vi "Send Command.vi"(7 "Config offset":u64 format="%x", 8 "error in (no error)":errorcluster, 9 "Command payload":u64 format="%x", 10 "Command number":T1, 11 "RP Instrument in":refnum<class "RP Instrument.lvclass">) -> (0 "error out":errorcluster, 3 "RP Instrument out":refnum<class "RP Instrument.lvclass">)   [LabVIEW 2024, in "RP Instrument.lvclass"]
uses:
  RP Instrument.lvclass
  RP Command.ctl
  RP Instrument.lvclass/RP Instrument.ctl
  RP Communicator/RP Communicator.lvclass
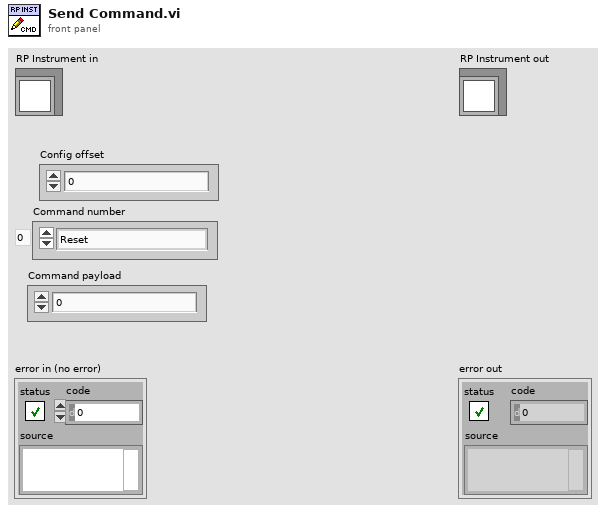
[diagram p1: front panel]
types:
  T1 = typedef "RP Command.ctl" = enum16{"Reset", "Read IDN", "Stop server", "Get status", "Get temperature", "Connect client", "Arm", "Software trigger", "Get whole buffer", "Get chunk", "System call", "Get config", "Set config", "Recieve data", "Recieve Calibartion", "Transmit data"}
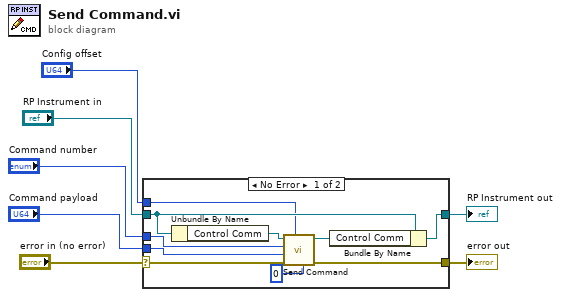
[diagram p0: block diagram]
diagram:
  n1 = case shown="No Error" "error in (no error)" {
    selector: "error in (no error)" -> [w11 w19]
    tunnel: [w10 w19] -> w6
    tunnel: [w16 w18] -> w4
    tunnel: "RP Instrument in" -> [w17 w18]
    tunnel: "Command number" -> [w14 _]
    tunnel: "Config offset" -> [w13 _]
    tunnel: "Command payload" -> [w12 _]
    frame No Error {
      n2 = Unbundle By Name(w17) -> ("Control Comm"=w15:refnum<class "RP Communicator.lvclass">)
      n3 = call-dynamic "Send Command.vi"("bytes to read"=0, "Config offset"=w13, "error in (no error)"=w11, "Command payload"=w12, "Command number"=w14, "RP Communicator in"=w15) -> ("error out"=w10:errorcluster, "RP Communicator out"=w9:refnum<class "RP Communicator.lvclass">)  [unwired: 3 in, 1 out]
      n4 = Bundle By Name(cluster=w17, "Control Comm"=w9) -> (w16:refnum<class "RP Instrument.lvclass">)
    }
    frame Error {
    }
  }
  "error out" <- w6
  "RP Instrument out" <- w4
